vi "Plot Grid (SubVI).vi"(9 "Polar Graph Attributes":T3, 10 "Draw Area Size":T2, 11 "new picture in":picture) -> (2 "grid measurements":T1, 3 "new picture out":picture)   [LabVIEW 2021]
uses:
  <vilib>/Utility/miscctls.llb/LVBoundsTypeDef.ctl
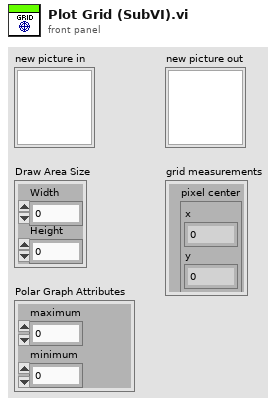
[diagram p1: front panel]
types:
  T1 = cluster{"pixel center":cluster{"x":i16, "y":i16}, "scale factors":cluster{"a":dbl, "b":dbl, "log?":bool}, "grid color":u32, "start angle":dbl, "end angle":dbl, "tick length":i16, "pixel radius":i32}
  T2 = typedef "LVBoundsTypeDef.ctl" = cluster{"Width":u32, "Height":u32}
  T3 = cluster{"maximum":dbl, "minimum":dbl, "clip to min":bool, "log?(F)":bool, "grid color":u32, "plot color":u32, "format and precision":cluster{"format":enum8{"Decimal", "Scientific", "Engineering", "Binary", "Octal", "Hex"}, "precision":u8}, "visible section":u16}
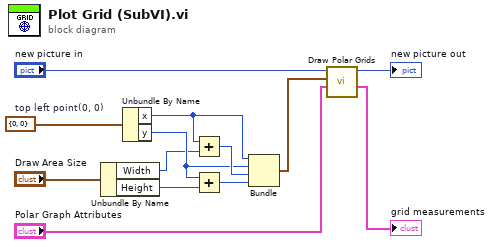
[diagram p0: block diagram]
diagram:
  w7 = cluster{"x":i16, "y":i16} {"x"=0, "y"=0}  # top left point(0, 0)
  n1 = Unbundle By Name("Draw Area Size") -> ("Width"=w1:u32, "Height"=w2:u32)
  n2 = Unbundle By Name(w7) -> ("x"=w3:i16, "y"=w4:i16)
  n3 = Add(x=w3, y=w1) -> (x+y=w5:u32)
  n4 = Add(x=w4, y=w2) -> (x+y=w6:u32)
  n5 = Bundle("x"=w3, "y"=w4, w5, w6) -> (w11:cluster{"x":i16, "y":i16, u32, u32})  [unwired: 1 in]
  n6 = call <vilib>:"Draw Polar Grids.vi"("polar attributes"="Polar Graph Attributes", "rect"=w11, "picture"="new picture in") -> ("grid measurements"=→"grid measurements":T1, "new picture"=→"new picture out":picture)  [unwired: 7 in]
